vi "ABB Test Heat run.vi"(10 "Measure":enum16{"Full Load", "Partial Load", "No Load"}(ring), 11 "Heat run Type":enum16{"Full Load", "Partial- & No-Load"}(ring)) -> ()   [LabVIEW 2017]
uses:
  Temp error msg.ctl
  <vilib>/Analysis/baseanly.llb/Mean (DBL).vi
  ABB global.vi
  <vilib>/Analysis/NI_AALBase.lvlib
panel:
  in  "Temp error":T1="Error: Temperature measurement "
  out "Additional Temperatures 2":string[][](table)
  out "Bearing Run readings":string[][](table)
  in  "Rated":T2
  in  "copying":string="Copying.."
  in  "copy to bearing":bool
  in  "Averaging":i32=1 min=1 max=1000
  in  "Smooth power\n    readings":bool
  in  "Reading Category":T3(ring)=enum."Wdg Temp"
  out "Power Readings":string[][](table)
  in  "Comments":string
  in  "Start":bool
  out "Type of Run":string
  out "Additional Temperatures":string[][](table)
  in  "Stabilitymessg":string="Thermal Stability reached"
  out "Time to Next reading":dbl(slide) scale=0.0..30.0 scale format="%#.1f"
  out "Start Time":dbl
  out "Temperatures":string[][](table)
  out "Readings":string[][](table)
  out "saved Readings":dbl[][](array[numeric])
  out "Serial number":string
  out "W.O number":string
  out "Norma 5000 Error":string
  in  "Record":bool
  out "Readings Table":string[][](table)
  in  "View":enum16{"Graph", "Readings"}(ring)
  out "Number readings":i32
  out "Status":enum16{"Stopped", "Running", "Finished"}(ring)
  out "Timedate":string
  in  "End test":bool
  in  "Read Mode":enum16{"Auto", "Manual"}(ring)
  in  "Exit":bool
  out "Temperature Trend":cluster{dbl[], "Best Linear Fit":dbl[]}[](graph)
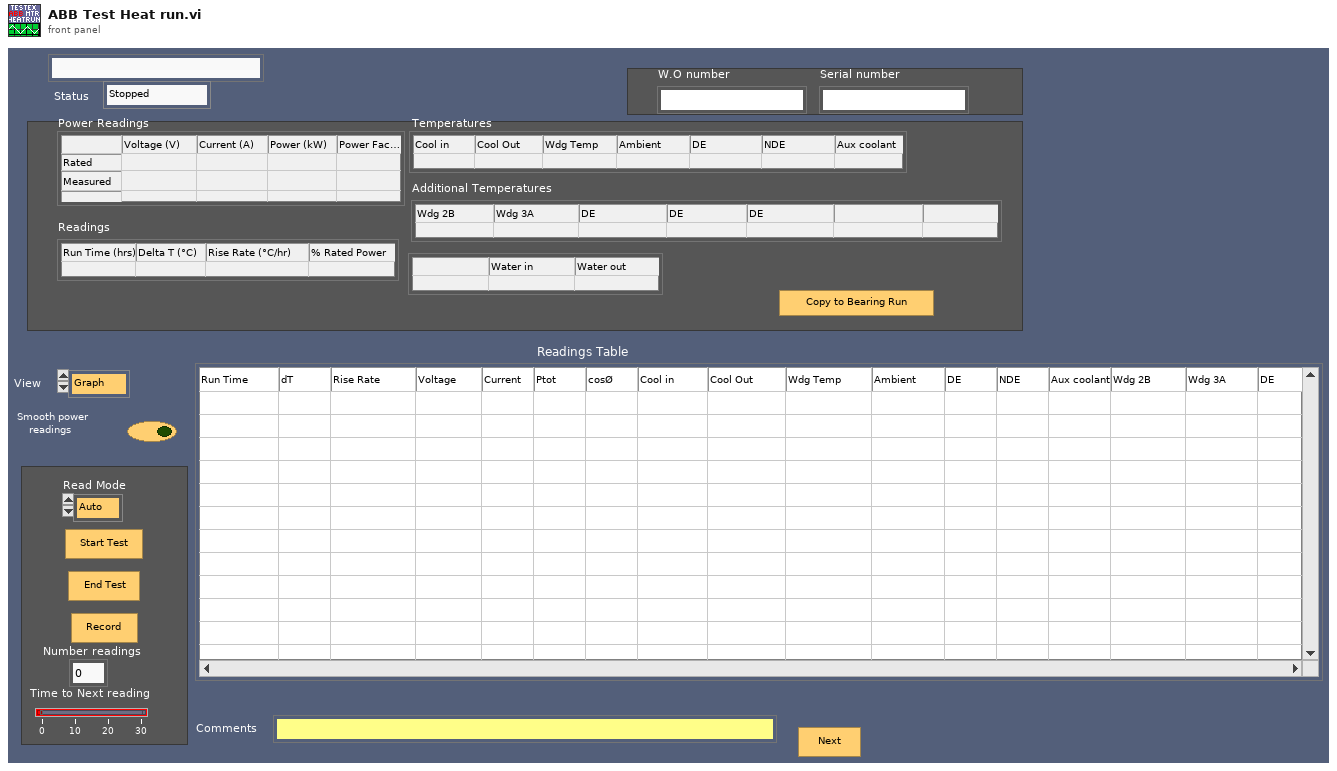
[diagram p1: front panel]
types:
  T1 = typedef "Temp error msg.ctl" = string
  T2 = cluster{"Voltage":dbl, "Current":dbl, "Power":dbl, "power factor":dbl}
  T3 = enum16{"None", "Cool in", "Cool Out", "Wdg Temp", "Ambient", "DE", "NDE", "Aux coolant"}
  T4 = enum16{"No load", "Locked Rotor", "Heat run", "NoLd heat run", "Partial heat run"}
  T5 = enum16{"Heat run", "Bearing run", "NoLd Heat Run", "Partial heat run"}
  T6 = cluster{"VT Primary":dbl, "VT Secondary":dbl, "CT  Primary":dbl, "CT Secondary":dbl, "Current Shunt":enum16{"Internal", "External"}, "Avg interval":dbl}
  T7 = cluster{"VT Primary":dbl, "VT Secondary":dbl, "CT  Primary":dbl, "CT Secondary":dbl, "Current Shunt":enum16{"Internal", "External"}, "Averaging interval (secs)":dbl}
  T8 = cluster{"Visa sesssion":refnum<visa-resource-name>, "error":errorcluster}
  T9 = cluster{"Simulate Norma":bool, "Norma 5000 Address":u8, "WebDaq IP Address":string, "Simulate cDAQ":bool}
  T10 = cluster{"Thermal Stability (deg/hr)":dbl, "Reading interval (mins)":dbl}
  T11 = cluster{"String":string, "String":string, "String":string, "String":string}
  T12 = cluster{"String":dbl, "String":dbl, "String":dbl, "String":dbl}
  T13 = cluster{"temp. alloc":i32[], "category":i32[], "Category names":string[], "Category none names":string[]}
  T14 = cluster{"V":dbl, "A":dbl, "W":dbl, "VA":dbl, "VAr":dbl, "Pf":dbl}
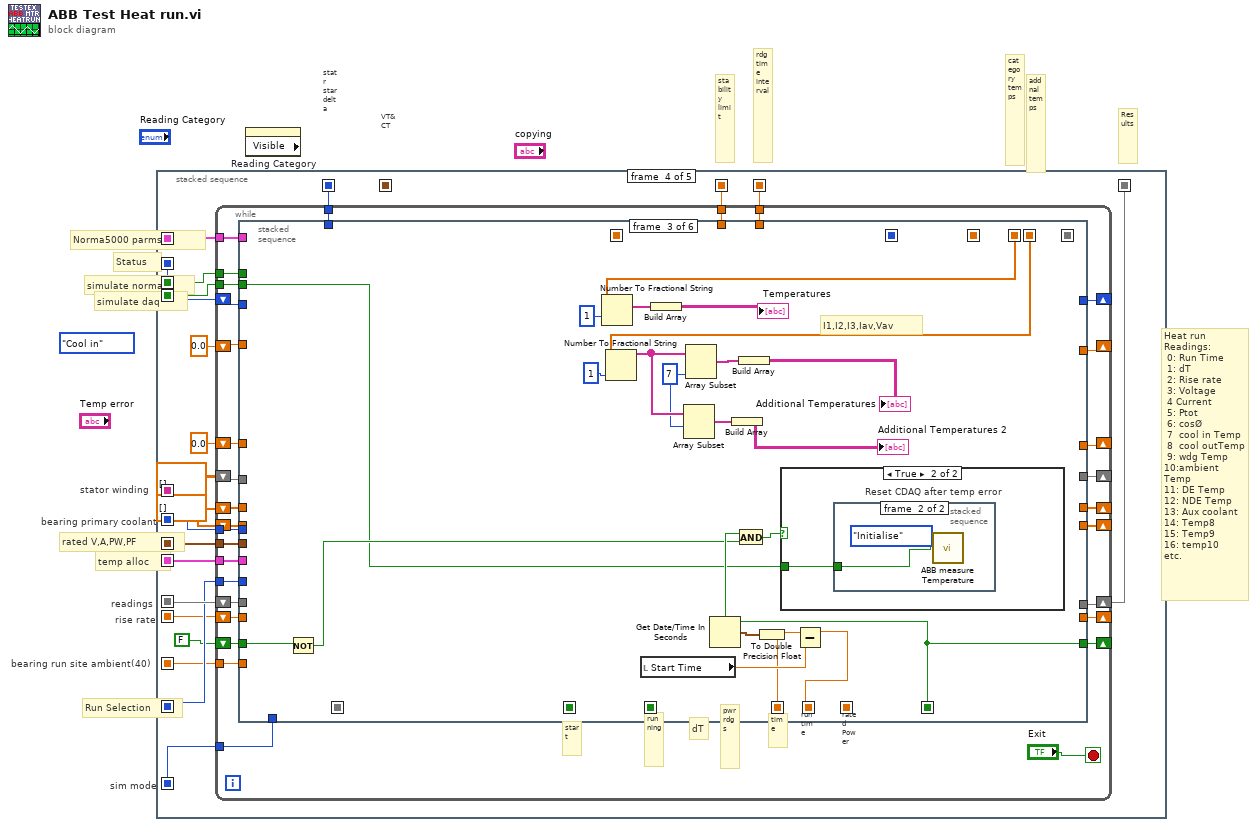
[diagram p0: block diagram]
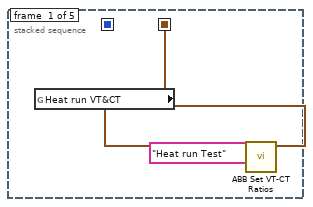
[diagram p2: hidden frame]
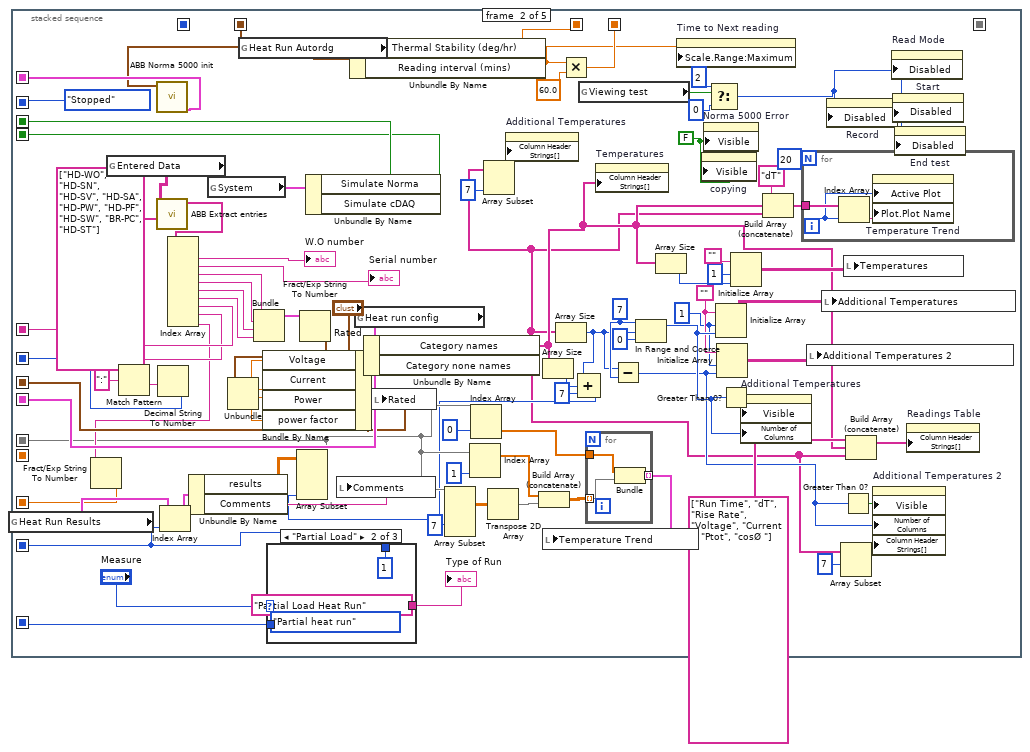
[diagram p3: hidden frame]
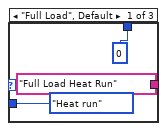
[diagram p4: hidden frame]
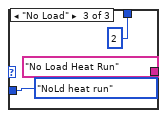
[diagram p5: hidden frame]
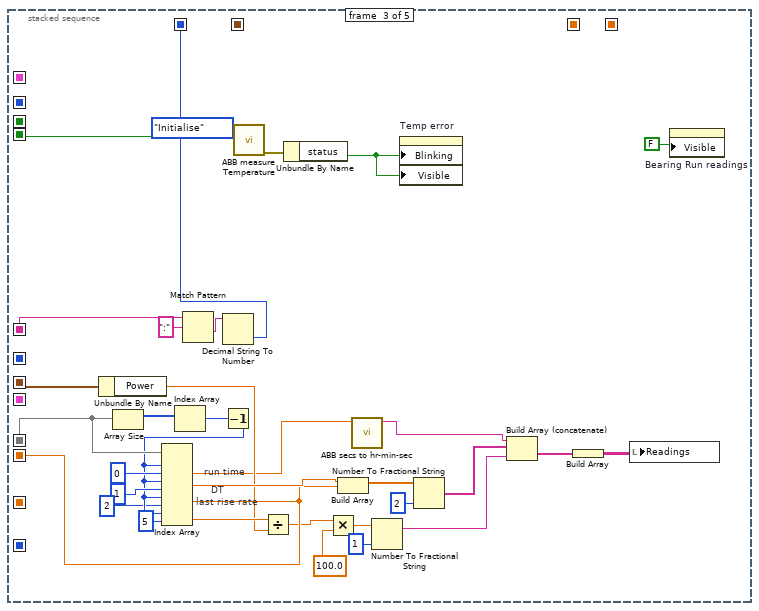
[diagram p6: hidden frame]
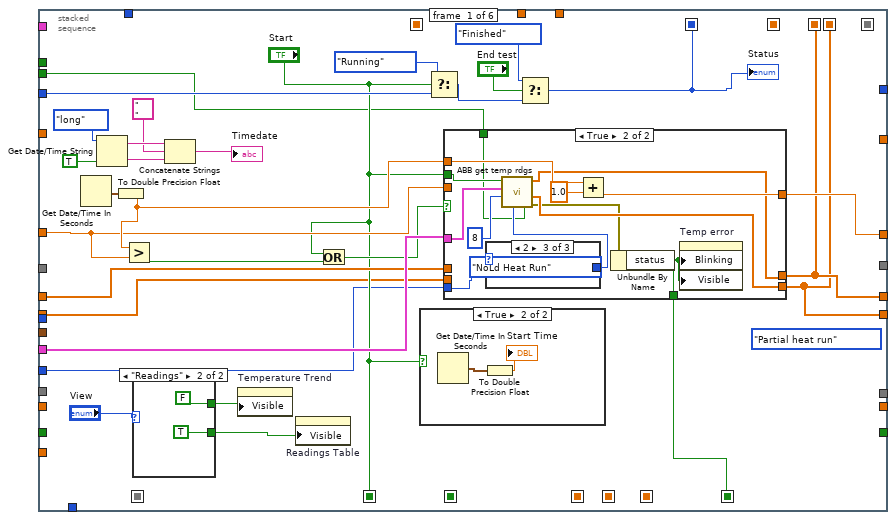
[diagram p7: hidden frame]
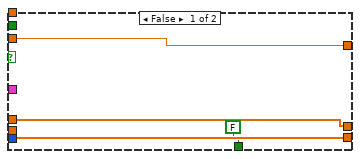
[diagram p9: hidden frame]
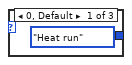
[diagram p10: hidden frame]
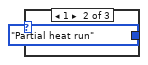
[diagram p11: hidden frame]
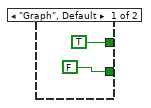
[diagram p12: hidden frame]
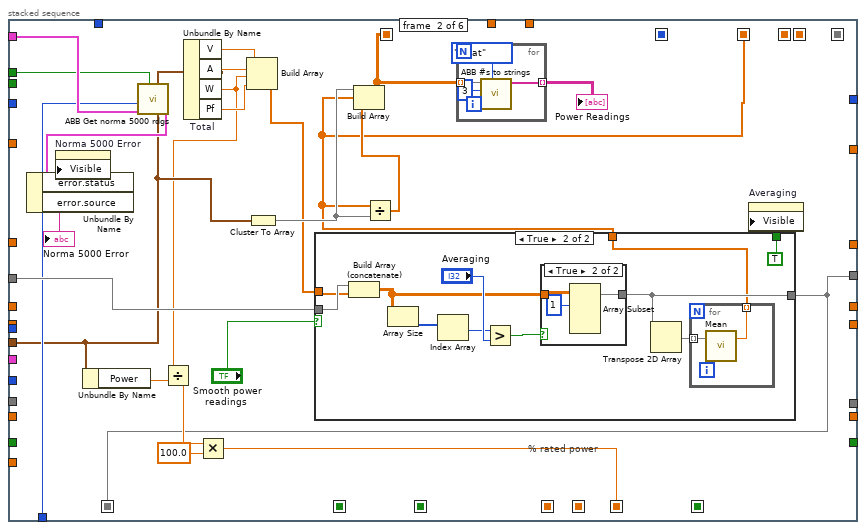
[diagram p13: hidden frame]
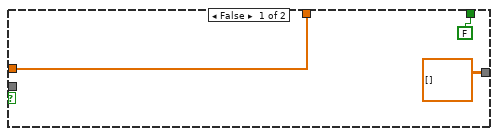
[diagram p14: hidden frame]
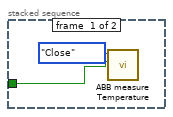
[diagram p17: hidden frame]
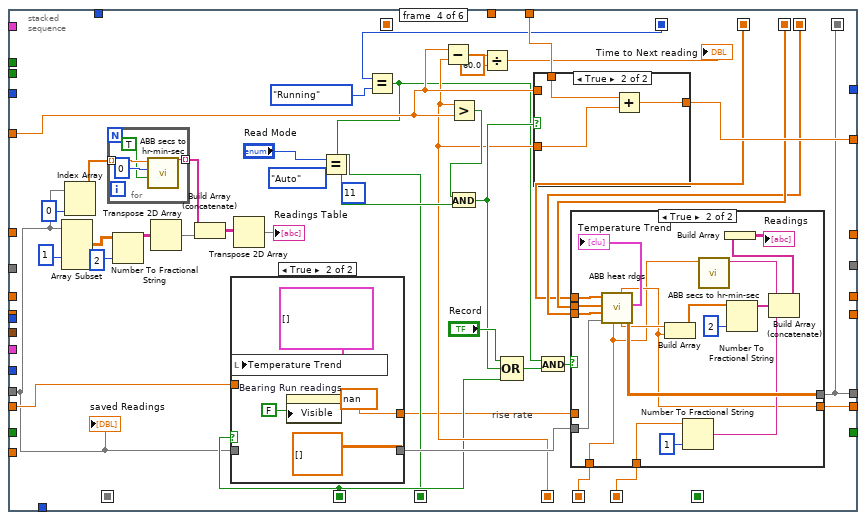
[diagram p18: hidden frame]
diagram:
  (unwired) T3."Cool in" ("Reading Category")
  # "bearing run site ambient(40)"
  # "bearing primary coolant"
  # "VT&CT"
  # "statr stardelta"
  # "stator winding"
  # "rise rate"
  # "readings"
  # "sim mode"
  # "simulate daq"
  # "addnal temps"
  # "category temps"
  # "Run Selection"
  # "stability limit"
  # "Results"
  # "rdg time interval"
  # "Heat run Readings:\n 0: Run Time\n 1: dT\n 2: Rise rate\n 3: Voltage\n 4 Current\n 5: Ptot\n 6: cosØ\n 7  cool in Temp\n 8  cool outTemp\n 9: wdg Temp\n10:ambient Temp\n11: DE Temp\n12: NDE Temp\n13: Aux coolant\n14: Temp8\n15: Temp9\n16: temp10\netc."
  # "temp alloc"
  # "rated V,A,PW,PF"
  # "simulate norma"
  # "Norma5000 parms"
  # "Status"
  n1 = stacked-sequence {
    seq-local: [_ enum16{"Stopped", "Running", "Finished"}."Stopped" ("Status") _ _ _] -> [_ _ _ w161 _]
    seq-local: [_ w90 _ _ _] -> [_ _ _ w160 w474]
    seq-local: [_ w88 _ _ _] -> [_ _ _ w159 w473]
    seq-local: [_ w38 _ _ _] -> [_ _ w129 w158 _]
    seq-local: [_ w7 _ _ _] -> [_ _ w138 w157 _]
    seq-local: [_ w53 _ _ _] -> [_ _ _ w155 _]
    seq-local: [_ w75 _ _ _] -> [_ _ _ w154 _]
    seq-local: [_ _ _ w152 _] -> [_ _ _ _ w471]
    seq-local: [_ w65 _ _ _] -> [_ _ _ w151 _]
    seq-local: [_ w47 _ _ _] -> [_ _ _ w148 w470]
    seq-local: [_ w51 _ _ _] -> [_ _ w110 w146 w467]
    seq-local: [_ w45 _ _ _] -> [_ _ _ w147 _]
    seq-local: [_ _ w132 _ _] -> [_ _ _ w145 _]
    seq-local: [_ w30 _ _ _] -> [_ _ w113 _ _]
    seq-local: [_ _ w112 _ _] -> [_ _ _ w144 _]
    seq-local: [w2 _ _ _ _] -> [_ w31 _ _ w469]
    seq-local: [_ w26 _ _ _] -> [_ _ _ w143 _]
    seq-local: [_ w24 _ _ _] -> [_ _ _ w142 _]
    frame #0 {
      n2 = global read "ABB global.vi" "Heat run VT&CT"() -> (w3:T6)
      n3 = call "ABB Set VT-CT Ratios.vi"("Test name"="Heat run Test", "VT and CT Ratios"=w3) -> ("VT and CT Ratios out"=w2:T7)  [unwired: 9 in]
    }
    frame #1 {
      w21 = 7 ("upper limit")
      w20 = ""
      w19 = 1 ("dimension size")
      w52 = FALSE ("Visible")
      n4 = global read "ABB global.vi" "Heat Run Results"() -> (w48:cluster{"results":dbl[][], "Comments":string}[])
      n5 = global read "ABB global.vi" "Entered Data"() -> (w71:string[][])
      n6 = call "ABB Norma 5000 init.vi"("VT and CT Ratios"=w31) -> ("norma 5000 parms out"=w90:T8)  [unwired: 10 in]
      n7 = call "ABB Extract entries.vi"("Entry IDs"=string[] ["HD-WO", "HD-SN", "HD-SV", "HD-SA", "HD-PW", "HD-PF", "HD-SW", "BR-PC", "HD-ST"], "Entry table in"=w71) -> ("Selected Entries"=w37:string[])  [unwired: 9 in]
      n8 = Index Array(array=w37) -> (element #1=→"W.O number":string, element #2=→"Serial number":string, element #3=w67:string, element #4=w55:string, element #5=w54:string, element #6=w56:string, element #7=w30:string, element #8=w27:string, element #9=w25:string)  [unwired: 9 in]
      n9 = Fract/Exp String To Number(string=w25) -> (number=w24:dbl)  [unwired: 3 in, 1 out]
      n10 = Match Pattern(string=w27, regular expression=":") -> (after substring=w28:string)  [unwired: 1 in, 3 out]
      n11 = Decimal String To Number(string=w28) -> (number=w26:i32)  [unwired: 2 in, 1 out]
      n12 = global read "ABB global.vi" "System"() -> (w89:T9)
      n13 = global read "ABB global.vi" "Heat Run Autordg"() -> (w87:T10)
      n14 = Bundle("String"=w67, "String"=w55, "String"=w54, "String"=w56) -> (w66:T11)  [unwired: 1 in]
      n15 = case shown="\"Partial Load\"" "Measure" {
        tunnel: ["Full Load Heat Run" "Partial Load Heat Run" "No Load Heat Run"] -> w50
        tunnel: [0 1 2] -> w47
        tunnel: [T4."Heat run" ("Simulate Mode") T4."Partial heat run" ("Simulate Mode") T4."NoLd heat run" ("Simulate Mode")] -> w45
        frame "Full Load", Default {
        }
        frame "Partial Load" {
        }
        frame "No Load" {
        }
      }
      "Type of Run" <- w50
      n16 = Index Array(array=w48, index=w47) -> (element=w61:cluster{"results":dbl[][], "Comments":string})
      n17 = Unbundle By Name(w61) -> ("results"=w8:dbl[][], "Comments"=w49:string)
      n18 = Fract/Exp String To Number(string=w66) -> (number=w43:T12)  [unwired: 3 in, 1 out]
      n19 = Unbundle(w43) -> ("String"=w42:dbl, "String"=w41:dbl, "String"=w40:dbl, "String"=w39:dbl)
      n20 = Bundle By Name(cluster="Rated", "Voltage"=w42, "Current"=w41, "Power"=w40, "power factor"=w39) -> (w38:T2)
      n21 = Unbundle By Name(w89) -> ("Simulate Norma"=w88:bool, "Simulate cDAQ"=w51:bool)
      n22 = local write "Comments"(w49) -> ()
      n23 = Unbundle By Name(w87) -> ("Thermal Stability (deg/hr)"=w65:dbl, "Reading interval (mins)"=w74:dbl)
      n24 = global read "ABB global.vi" "Heat run config"() -> (w53:T13)
      n25 = Unbundle By Name(w53) -> ("Category names"=w5:string[], "Category none names"=w4:string[])
      n26 = local write "Rated"(w38) -> ()
      n27 = Array Subset(array=w4, length=7) -> (w15:string[])  [unwired: 1 in]
      n28 = property on="Additional Temperatures" class="Tbl (strict)"("Column Header Strings[]"=w15) -> ()  [unwired: 2 in, 2 out]
      n29 = Array Size(array=w5) -> (size(s)=w11:i32)
      n30 = Array Size(array=w4) -> (size(s)=w10:i32)
      n31 = Multiply(x=w74, y=60.0) -> (x*y=w75:dbl)
      n32 = Compound Arithmetic op=ADD(w10, w11, 7 ("value")) -> (w6:i32)
      n33 = Array Subset(array=w8, length (col)=w6) -> (w7:dbl[][])  [unwired: 3 in]
      n34 = Array Subset(array=w7, index (col)=7 ("index")) -> (w78:dbl[][])  [unwired: 3 in]
      n35 = Index Array(array=w7, index (col)=1 ("disabled index (col)")) -> (element=w32:dbl[])  [unwired: 1 in]
      n36 = Index Array(array=w7, index (col)=0 ("disabled index (col)")) -> (element=w80:dbl[])  [unwired: 1 in]
      n37 = Transpose 2D Array(2D array=w78) -> (transposed array=w77:dbl[][])
      n38 = Build Array (concatenate)(w32, w77) -> (w33:dbl[][])
      n39 = global read "ABB global.vi" "Viewing test"() -> (w60:bool)
      n40 = for {
        tunnel: w80 -> [w103]
        tunnel: w33 -> [w102] mode=indexing
        tunnel: [w101] -> w76 mode=indexing
        n41 = Bundle(w103, w102) -> (w101:cluster{dbl[], dbl[]})  [unwired: 1 in]
      }
      n42 = local write "Temperature Trend"(w76) -> ()
      n43 = property on="Temperatures" class="Tbl (strict)"("Column Header Strings[]"=w5) -> ()  [unwired: 2 in, 2 out]
      n44 = Subtract(x=w10, y=w21) -> (x-y=w16:i32)
      n45 = In Range and Coerce(upper limit=w21, x=w10, lower limit=0) -> (coerced(x)=w23:i32)  [unwired: 1 out]
      n46 = Array Size(array=w5) -> (size(s)=w85:i32)
      n47 = property on="Time to Next reading" class="Slide (strict)"("Scale.Range:Maximum"=w74) -> ()  [unwired: 2 in, 2 out]
      n48 = property on="copying" class="Str"("Visible"=w52) -> ()  [unwired: 2 in, 2 out]
      n49 = property on="Norma 5000 Error" class="Str"("Visible"=w52) -> ()  [unwired: 2 in, 2 out]
      n50 = Select(t=2, s=w60, f=0) -> (s? t:f=w57:i32)
      n51 = Initialize Array(w20, w19, w23) -> (w64:string[][])
      n52 = Initialize Array(w20, w19, w16) -> (w18:string[][])
      n53 = Greater Than 0?(x=w23) -> (x > 0?=w63:bool)
      n54 = Initialize Array("", 1 ("dimension size"), w85) -> (w83:string[][])
      n55 = property on="Additional Temperatures" class="Tbl (strict)"("Visible"=w63, "Number of Columns"=w23) -> ()  [unwired: 2 in, 2 out]
      n56 = Build Array (concatenate)("dT", w5, w4) -> (w36:string[])
      n57 = for {
        N: 20 -> [_]
        tunnel: w36 -> [w106]
        i -> [w105]
        n58 = Index Array(array=w106, index=w105) -> (element=w104:string)
        n59 = property on="Temperature Trend" class="XYGraph (strict)"("Active Plot"=w105, "Plot.Plot Name"=w104) -> ()  [unwired: 2 in, 2 out]
      }
      n60 = local write "Additional Temperatures 2"(w18) -> ()
      n61 = local write "Additional Temperatures"(w64) -> ()
      n62 = property on="Record" class="Bool"("Disabled"=w57) -> ()  [unwired: 2 in, 2 out]
      n63 = Array Subset(array=w4, index=7) -> (w12:string[])  [unwired: 1 in]
      n64 = Greater Than 0?(x=w16) -> (x > 0?=w17:bool)
      n65 = local write "Temperatures"(w83) -> ()
      n66 = Build Array (concatenate)(string[] ["Run Time", "dT", "Rise Rate", "Voltage", "Current ", "Ptot", "cosØ "], w5, w4) -> (w72:string[])
      n67 = property on="Additional Temperatures 2" class="Tbl (strict)"("Visible"=w17, "Number of Columns"=w16, "Column Header Strings[]"=w12) -> ()  [unwired: 2 in, 2 out]
      n68 = property on="Read Mode" class="Enum (strict)"("Disabled"=w57) -> ()  [unwired: 2 in, 2 out]
      n69 = property on="Start" class="Bool"("Disabled"=w57) -> ()  [unwired: 2 in, 2 out]
      n70 = property on="End test" class="Bool"("Disabled"=w57) -> ()  [unwired: 2 in, 2 out]
      n71 = property on="Readings Table" class="Tbl (strict)"("Column Header Strings[]"=w72) -> ()  [unwired: 2 in, 2 out]
    }
    frame #2 {
      # "DT"
      # "run time"
      # "last rise rate"
      n72 = Unbundle By Name(w129) -> ("Power"=w128:dbl)
      n73 = Array Size(array=w138) -> (size(s)=w140:i32[])
      n74 = Index Array(array=w140) -> (element=w139:i32)  [unwired: 1 in]
      n75 = Match Pattern(string=w113, regular expression=":") -> (after substring=w114:string)  [unwired: 1 in, 3 out]
      n76 = Decimal String To Number(string=w114) -> (number=w112:i32)  [unwired: 2 in, 1 out]
      n77 = Decrement(x=w139) -> (x-1=w135:i32)
      n78 = Index Array(array=w138, index (row) #1=w135, index (col) #1=0, index (row) #2=w135, index (col) #2=1 ("disabled index (col)"), index (row) #3=w135, index (col) #3=2 ("disabled index (col)"), index (row) #4=w135, index (col) #4=5 ("disabled index (col)")) -> (element #1=w117:dbl, element #2=w134:dbl, element #3=w132:dbl, element #4=w130:dbl)
      n79 = call "ABB measure Temperature.vi"("Simulate"=w110, "Mode"=enum16{"Initialise", "Read", "Close"}."Initialise") -> ("error out"=w108:errorcluster)  [unwired: 7 in, 2 out]
      n80 = Divide(x=w130, y=w128) -> (x/y=w125:dbl)
      n81 = Unbundle By Name(w108) -> ("status"=w107:bool)
      n82 = Multiply(x=w125, y=100.0) -> (x*y=w119:dbl)
      n83 = Build Array(w134, w132) -> (w127:dbl[])
      n84 = call "ABB secs to hr-min-sec.vi"("Seconds"=w117) -> ("hr:min:secs"=w116:string)  [unwired: 10 in]
      n85 = Number To Fractional String(number=w119, precision (6)=i16 1) -> (F-format string=w122:string)  [unwired: 2 in]
      n86 = property on="Temp error" class="Str (strict)"("Blinking"=w107, "Visible"=w107) -> ()  [unwired: 2 in, 2 out]
      n87 = Number To Fractional String(number=w127, precision (6)=i16 2) -> (F-format string=w123:string[])  [unwired: 2 in]
      n88 = Build Array (concatenate)(w116, w123, w122) -> (w121:string[])
      n89 = Build Array(w121) -> (w120:string[][])
      n90 = local write "Readings"(w120) -> ()
      n91 = property on="Bearing Run readings" class="Tbl (strict)"("Visible"=FALSE) -> ()  [unwired: 2 in, 2 out]
    }
    frame #3 {
      w150 = dbl[] []
      n92 = while {
        shift-right: [w190] -> _
        shift-left: w161 -> [w191]
        tunnel: w160 -> [w189]
        tunnel: w159 -> [w188]
        tunnel: w158 -> [w187]
        shift-right: [w185] -> w152
        shift-left: w157 -> [w186]
        shift-right: [w182] -> _
        shift-left: 0.0 -> [w184]
        shift-right: [w183] -> _
        shift-left: w150 -> [w180]
        tunnel: w155 -> [w181]
        tunnel: w154 -> [w179]
        shift-right: [w177] -> _
        shift-left: 0.0 -> [w178]
        tunnel: w151 -> [w176]
        shift-right: [w174] -> _
        shift-left: w150 -> [w175]
        shift-right: [w172] -> _
        shift-left: dbl[][] [] -> [w173]
        tunnel: w148 -> [w171]
        tunnel: w147 -> [w170]
        tunnel: w146 -> [w169]
        shift-right: [w168] -> _
        shift-left: w145 -> [w167]
        tunnel: w144 -> [w166]
        tunnel: w143 -> [w165]
        tunnel: w142 -> [w164]
        shift-right: [w163] -> _
        shift-left: FALSE -> [w162]
        stop <- "Exit" stop-if-true
        # "run time"
        # "% rated Power"
        # "running"
        # "time"
        # "dT"
        # "pwr rdgs"
        # "start"
        n93 = stacked-sequence {
          seq-local: ["Start" _ _ _ _ _] -> [_ _ _ w346 _ _]
          seq-local: [_ w258 _ _ _ _] -> [_ _ _ w340 _ _]
          seq-local: [_ _ w316 _ _ _] -> [_ _ _ w351 _ _]
          seq-local: [w200 _ _ _ _ _] -> [_ _ _ w344 w402 _]
          seq-local: [w199 _ _ _ _ _] -> [_ _ w314 w343 _ _]
          seq-local: [_ _ _ w342 _ _] -> [_ _ _ _ w408 _]
          seq-local: [w196 _ _ _ _ _] -> [_ _ w312 w341 _ _]
          seq-local: [_ w262 _ _ _ _] -> [_ _ _ _ _ _]
          seq-local: [_ _ _ w339 _ _] -> [_ _ _ _ w401 w422]
          seq-local: [_ w250 _ _ _ _] -> [_ _ _ w337 _ _]
          seq-local: [_ w249 _ _ _ _] -> [_ _ _ _ _ _]
          seq-local: [_ _ w309 _ _ _] -> [_ _ _ w338 _ _]
          seq-local: [w193 _ _ _ _ _] -> [_ _ w303 _ _ _]
          tunnel: w191 -> [w216 _ _ _ w412 _]
          tunnel: [_ _ _ _ w402 _] -> w190
          tunnel: w189 -> [_ w274 _ _ _ _]
          tunnel: w188 -> [_ w270 _ _ _ _]
          tunnel: w187 -> [_ w255 _ _ _ _]
          tunnel: w186 -> [_ _ _ w332 w416 _]
          tunnel: [_ _ _ w339 _ _] -> w185
          tunnel: w184 -> [w206 _ _ _ _ _]
          tunnel: [w199 _ _ _ _ _] -> w183
          tunnel: [w205 _ _ _ _ _] -> w182
          tunnel: w181 -> [w204 _ _ _ _ _]
          tunnel: w180 -> [w203 _ _ _ _ _]
          tunnel: w179 -> [_ _ _ w362 _ _]
          tunnel: w178 -> [_ _ _ w352 _ _]
          tunnel: [_ _ _ w361 _ _] -> w177
          tunnel: w176 -> [_ _ _ _ w415 _]
          tunnel: w175 -> [w197 _ _ _ _ _]
          tunnel: [w196 _ _ _ _ _] -> w174
          tunnel: w173 -> [_ w261 _ _ _ _]
          tunnel: [_ w249 _ _ _ _] -> w172
          tunnel: w171 -> [w195 _ _ _ _ _]
          tunnel: w170 -> [_ w256 _ _ _ _]
          tunnel: w169 -> [w194 _ w299 _ _ _]
          tunnel: [_ _ _ w336 _ _] -> w168
          tunnel: w167 -> [_ _ _ w335 w404 _]
          tunnel: w166 -> [_ _ _ _ _ _]
          tunnel: w165 -> [_ _ _ _ _ w421]
          tunnel: w164 -> [_ _ _ _ _ w420]
          tunnel: [_ _ w303 _ _ _] -> w163
          tunnel: w162 -> [_ _ w302 _ _ _]
          frame #0 {
            (unwired) T5."Partial heat run" ("sim type")
            n94 = Get Date/Time In Seconds() -> (seconds since 1Jan1904=w208:timestamp)
            n95 = Get Date/Time String(date format (0)=enum16{"short", "long", "abbreviated"}."long", want seconds? (F)=TRUE) -> (date string=w220:string, time string=w219:string)  [unwired: 1 in]
            n96 = To Double Precision Float(number=w208) -> (double precision float=w207:dbl)
            n97 = Greater?(x=w207, y=w206) -> (0:w202:bool)
            n98 = case shown="\"Readings\"" "View" {
              tunnel: [TRUE FALSE] -> w210
              tunnel: [FALSE TRUE] -> w209
              frame "Graph", Default {
              }
              frame "Readings" {
              }
            }
            n99 = Concatenate Strings(w220, "   ", w219) -> (→"Timedate":string)
            n100 = property on="Temperature Trend" class="XYGraph (strict)"("Visible"=w210) -> ()  [unwired: 2 in, 2 out]
            n101 = property on="Readings Table" class="Tbl (strict)"("Visible"=w209) -> ()  [unwired: 2 in, 2 out]
            n102 = Or(x="Start", y=w202) -> (x .or. y?=w201:bool)
            n103 = case shown="True" "Start" {
              frame False {
              }
              frame True {
                n104 = Get Date/Time In Seconds() -> (seconds since 1Jan1904=w224:timestamp)
                n105 = To Double Precision Float(number=w224) -> (double precision float=→"Start Time":dbl)
              }
            }
            n106 = Select(t=enum16{"Stopped", "Running", "Finished"}."Running", s="Start", f=w216) -> (s? t:f=w214:enum16{"Stopped", "Running", "Finished"})
            n107 = case shown="True" w201 {
              tunnel: w207 -> [_ w241]
              tunnel: [w228 w239] -> w205
              tunnel: w206 -> [w228 _]
              tunnel: w194 -> [_ w231]
              tunnel: w204 -> [_ w237]
              tunnel: [w227 w236] -> w199
              tunnel: w203 -> [w227 _]
              tunnel: "Start" -> [_ w238]
              tunnel: w197 -> [w226 _]
              tunnel: [w226 w235] -> w196
              tunnel: w195 -> [_ w233]
              tunnel: [FALSE ("status") w229] -> w193
              frame False {
              }
              frame True {
                n108 = case shown="2" w233 {
                  tunnel: [T5."Heat run" ("sim type") T5."Partial heat run" ("sim type") T5."NoLd Heat Run" ("sim type")] -> w232
                  frame 0, Default {
                  }
                  frame 1 {
                  }
                  frame 2 {
                  }
                }
                n109 = call "ABB get temp rdgs.vi"("Sim daq"=w231, "sim type"=w232, "# categories"=8, "run config"=w237, "start"=w238) -> ("error out"=w230:errorcluster, "Category none rdgs"=w235:dbl[], "Category rdgs"=w236:dbl[])  [unwired: 3 in, 1 out]
                n110 = Add(x=w241, y=1.0) -> (x+y=w239:dbl)
                n111 = Unbundle By Name(w230) -> ("status"=w229:bool)
                n112 = property on="Temp error" class="Str (strict)"("Blinking"=w229, "Visible"=w229) -> ()  [unwired: 2 in, 2 out]
              }
            }
            n113 = Select(t=enum16{"Stopped", "Running", "Finished"}."Finished", s="End test", f=w214) -> (s? t:f=w200:enum16{"Stopped", "Running", "Finished"})
            "Status" <- w200
          }
          frame #1 {
            # "% rated power"
            n114 = Unbundle By Name(w255) -> ("Power"=w254:dbl)
            n115 = call "ABB Get norma 5000 rdgs.vi"("Rated"=w255, "simulate"=w270, "norma 5000 parms in"=w274, "Simulate Mode"=w256) -> ("norma 5000 parms out"=w271:T8, "Total"=w269:T14)  [unwired: 3 in, 3 out]
            n116 = Unbundle By Name(w271) -> ("error.status"=w273:bool, "error.source"=→"Norma 5000 Error":string)
            n117 = property on="Norma 5000 Error" class="Str"("Visible"=w273) -> ()  [unwired: 2 in, 2 out]
            n118 = Unbundle By Name "Total"(w269) -> ("V"=w265:dbl, "A"=w264:dbl, "W"=w253:dbl, "Pf"=w263:dbl)
            n119 = Divide(x=w253, y=w254) -> (x/y=w252:dbl)
            n120 = Multiply(x=w252, y=100.0) -> (x*y=w250:dbl)
            n121 = Build Array(w265, w264, w253, w263) -> (w259:dbl[])
            n122 = Cluster To Array(cluster=w255) -> (array=w266:dbl[])
            n123 = case shown="True" "Smooth power\n    readings" {
              tunnel: w261 -> [_ w282]
              tunnel: w259 -> [w277 w281]
              tunnel: [dbl[][] [] w284] -> w249
              tunnel: [w277 w283] -> w258
              tunnel: [FALSE TRUE] -> w257
              frame False {
              }
              frame True {
                n124 = Build Array (concatenate)(w282, w281) -> (w285:dbl[][])
                n125 = Array Size(array=w285) -> (size(s)=w288:i32[])
                n126 = Index Array(array=w288) -> (element=w278:i32)  [unwired: 1 in]
                n127 = Greater?(x=w278, y="Averaging") -> (0:w286:bool)
                n128 = case shown="True" w286 {
                  tunnel: w285 -> [w291 w294]
                  tunnel: [w291 w293] -> w284
                  frame False {
                  }
                  frame True {
                    n129 = Array Subset(array=w294, index (row)=1 ("index")) -> (w293:dbl[][])  [unwired: 3 in]
                  }
                }
                n130 = Transpose 2D Array(2D array=w284) -> (transposed array=w280:dbl[][])
                n131 = for {
                  tunnel: w280 -> [w290] mode=indexing
                  tunnel: [w289] -> w283 mode=indexing
                  n132 = call-poly <vilib>:"Mean.vi"("X"=w290) -> ("mean"=w289:dbl)  [unwired: 1 out]
                }
              }
            }
            n133 = Divide(x=w258, y=w266) -> (x/y=w267:dbl[])
            n134 = Build Array(w266, w258, w267) -> (w262:dbl[][])
            n135 = for {
              tunnel: w262 -> [w298] mode=indexing
              tunnel: [w295] -> w268 mode=indexing
              n136 = call "ABB #s to strings.vi"("# type"=enum16{"Float", "Relative time HH:MM"}."Float", "Precision"=3, "Numbers in"=w298) -> ("Strings out"=w295:string[])  [unwired: 8 in]
            }
            "Power Readings" <- w268
            n137 = property on="Averaging" class="DigNum (strict)"("Visible"=w257) -> ()  [unwired: 2 in, 2 out]
          }
          frame #2 {
            w304 = 7 ("length")
            # "I1,I2,I3,Iav,Vav"
            n138 = Not(x=w302) -> (.not. x?=w300:bool)
            n139 = Number To Fractional String(number=w314, precision (6)=i16 1) -> (F-format string=w313:string[])  [unwired: 2 in]
            n140 = Number To Fractional String(number=w312, precision (6)=i16 1) -> (F-format string=w307:string[])  [unwired: 2 in]
            n141 = local read "Start Time"() -> (w317:dbl)
            n142 = Build Array(w313) -> (→"Temperatures":string[][])
            n143 = Array Subset(array=w307, index=w304) -> (w305:string[])  [unwired: 1 in]
            n144 = Array Subset(array=w307, length=w304) -> (w308:string[])  [unwired: 1 in]
            n145 = Get Date/Time In Seconds() -> (seconds since 1Jan1904=w318:timestamp)
            n146 = Build Array(w305) -> (→"Additional Temperatures 2":string[][])
            n147 = And(x=w303, y=w300) -> (x .and. y?=w301:bool)
            n148 = Build Array(w308) -> (→"Additional Temperatures":string[][])
            n149 = To Double Precision Float(number=w318) -> (double precision float=w316:dbl)
            n150 = case shown="True" w301 {
              tunnel: w299 -> [_ w320]
              frame False {
              }
              frame True {
                # "Reset CDAQ after temp error"
                n151 = stacked-sequence {
                  tunnel: w320 -> [w321 w323]
                  frame #0 {
                    n152 = call "ABB measure Temperature.vi"("Simulate"=w321, "Mode"=enum16{"Initialise", "Read", "Close"}."Close") -> ()  [unwired: 7 in, 3 out]
                  }
                  frame #1 {
                    n153 = call "ABB measure Temperature.vi"("Simulate"=w323, "Mode"=enum16{"Initialise", "Read", "Close"}."Initialise") -> ()  [unwired: 7 in, 3 out]
                  }
                }
              }
            }
            n154 = Subtract(x=w316, y=w317) -> (x-y=w309:dbl)
          }
          frame #3 {
            (unwired) 11 ("index")
            # "rise rate"
            n155 = Array Subset(array=w332, index (col)=1 ("index")) -> (w333:dbl[][])  [unwired: 3 in]
            n156 = Index Array(array=w332, index (col)=0 ("disabled index (col)")) -> (element=w331:dbl[])  [unwired: 1 in]
            n157 = for {
              tunnel: w331 -> [w368] mode=indexing
              tunnel: [w366] -> w327 mode=indexing
              n158 = call "ABB secs to hr-min-sec.vi"("round off secs"=TRUE, "Precision"=i16 0, "Seconds"=w368) -> ("hr:min:secs"=w366:string)  [unwired: 8 in]
            }
            n159 = Number To Fractional String(number=w333, precision (6)=i16 2) -> (F-format string=w347:string[][])  [unwired: 2 in]
            n160 = Transpose 2D Array(2D array=w347) -> (transposed array=w326:string[][])
            n161 = Build Array (concatenate)(w327, w326) -> (w330:string[][])
            n162 = case shown="True" w346 {
              tunnel: w332 -> [w374 _]
              tunnel: [w374 dbl[][] []] -> w355
              tunnel: w335 -> [w373 _]
              tunnel: [w373 nan] -> w334
              frame False {
              }
              frame True {
                n163 = local write "Temperature Trend"(cluster{dbl[], "Best Linear Fit":dbl[]}[] [] ("Temperature Trend")) -> ()
                n164 = property on="Bearing Run readings" class="Tbl (strict)"("Visible"=FALSE) -> ()  [unwired: 2 in, 2 out]
              }
            }
            n165 = Transpose 2D Array(2D array=w330) -> (transposed array=→"Readings Table":string[][])
            n166 = Equal?(x="Read Mode", y=enum16{"Auto", "Manual"}."Auto") -> (x = y?=w358:bool)
            n167 = Equal?(x=w344, y=enum16{"Stopped", "Running", "Finished"}."Running" ("x")) -> (x = y?=w342:bool)
            n168 = Subtract(x=w352, y=w351) -> (x-y=w350:dbl)
            n169 = Greater?(x=w351, y=w352) -> (0:w357:bool)
            n170 = And(x=w357, y=w358) -> (x .and. y?=w356:bool)
            n171 = Divide(x=w350, y=60.0) -> (x/y=→"Time to Next reading":dbl)
            n172 = Compound Arithmetic op=OR("Record", w356, w346) -> (w353:bool)
            n173 = case shown="True" w356 {
              tunnel: w362 -> [_ w371]
              tunnel: w351 -> [_ w372]
              tunnel: [w369 w370] -> w361
              tunnel: w352 -> [w369 _]
              frame False {
              }
              frame True {
                n174 = Add(x=w371, y=w372) -> (x+y=w370:dbl)
              }
            }
            n175 = And(x=w342, y=w353) -> (x .and. y?=w354:bool)
            n176 = case shown="True" w354 {
              tunnel: w355 -> [w380 w395]
              tunnel: [w380 w394] -> w339
              tunnel: w340 -> [_ w398]
              tunnel: w343 -> [_ w397]
              tunnel: w341 -> [_ w393]
              tunnel: w338 -> [_ w381]
              tunnel: w337 -> [_ w382]
              tunnel: [w379 w383] -> w336
              tunnel: w334 -> [w379 _]
              frame False {
              }
              frame True {
                n177 = call "ABB heat rdgs.vi"("Run Time"=w381, "Readings in"=w395, "Addnl temps"=w393, "temperatures"=w397, "power"=w398) -> ("Readings out"=w394:dbl[][], "Temperature trend"=→"Temperature Trend":cluster{dbl[], dbl[]}[], "dT"=w386:dbl, "rise rate"=w383:dbl)  [unwired: 3 in]
                n178 = Build Array(w386, w383) -> (w390:dbl[])
                n179 = Number To Fractional String(number=w382, precision (6)=i16 1) -> (F-format string=w384:string)  [unwired: 2 in]
                n180 = call "ABB secs to hr-min-sec.vi"("Seconds"=w381) -> ("hr:min:secs"=w388:string)  [unwired: 10 in]
                n181 = Number To Fractional String(number=w390, precision (6)=i16 2) -> (F-format string=w392:string[])  [unwired: 2 in]
                n182 = Build Array (concatenate)(w388, w392, w384) -> (w391:string[])
                n183 = Build Array(w391) -> (→"Readings":string[][])
              }
            }
            "saved Readings" <- w332
          }
          frame #4 {
            n184 = Array Size(array=w416) -> (size(s)=w419:i32[])
            n185 = Index Array(array=w419) -> (element=w418:i32)  [unwired: 1 in]
            n186 = Not Equal?(x=w412, y=enum16{"Stopped", "Running", "Finished"}."Stopped") -> (x != y?=w410:bool)
            n187 = Greater?(x=w418, y=2) -> (0:w413:bool)
            n188 = Absolute Value(x=w404) -> (abs(x)=w403:dbl)
            n189 = Less?(x=w403, y=w415) -> (x < y?=w414:bool)
            n190 = Wait Until Next ms Multiple(millisecond multiple=u32 200) -> ()  [unwired: 1 out]
            n191 = Compound Arithmetic op=AND(w414, w410, w413) -> (w407:bool)
            n192 = And(x=w407, y=w408) -> (x .and. y?=w406:bool)
            n193 = Select(t=enum16{"Stopped", "Running", "Finished"}."Finished", s=w406, f=w402) -> ()  [unwired: 1 out]
            n194 = property on="Stabilitymessg" class="Str"("Visible"=w407, "Blinking"=w407) -> ()  [unwired: 2 in, 2 out]
            n195 = property on="Time to Next reading" class="Slide (strict)"("Visible"=w408) -> ()  [unwired: 2 in, 2 out]
            n196 = Array Size(array=w401) -> (size(s)=w400:i32[])
            n197 = Index Array(array=w400) -> (element=→"Number readings":i32)  [unwired: 1 in]
          }
          frame #5 {
            n198 = case shown="True" "copy to bearing" {
              tunnel: w422 -> [_ w426]
              tunnel: w421 -> [_ w425]
              tunnel: w420 -> [_ w424]
              frame False {
              }
              frame True {
                n199 = stacked-sequence {
                  tunnel: w426 -> [_ w456 _]
                  tunnel: w425 -> [_ w448 _]
                  tunnel: w424 -> [_ w442 _]
                  frame #0 {
                    w427 = TRUE ("Visible")
                    n200 = property on="copying" class="Str"("Visible"=w427) -> ()  [unwired: 2 in, 2 out]
                    n201 = property on="Bearing Run readings" class="Tbl (strict)"("Visible"=w427) -> ()  [unwired: 2 in, 2 out]
                  }
                  frame #1 {
                    w430 = 2
                    (unwired) nan
                    # "Bearing run Readings:\n 0: Run Time\n 1: DE Rise\n 2: NDE Rise\n 3:DT\n4: Cool In\n5:Ambient\n6:DE Temp\n8: NDE Temp\n9: temp\netc."
                    # "Ambient"
                    # "Aux coolant"
                    # "NDE"
                    # "DE"
                    # "Run time"
                    n202 = Index Array(array=w456, index (col) #1=0 ("disabled index (col)"), index (col) #2=11 ("index (col)"), index (col) #3=12 ("index (col)"), index (col) #4=13 ("index (col)"), index (col) #5=10 ("index (col)")) -> (element #1=w450:dbl[], element #2=w445:dbl[], element #3=w444:dbl[], element #4=w447:dbl[], element #5=w446:dbl[])  [unwired: 5 in]
                    n203 = Build Array(w447, w446, w445, w444) -> (w443:dbl[][])
                    n204 = Transpose 2D Array(2D array=w443) -> (transposed array=w431:dbl[][])
                    n205 = for {
                      tunnel: w450 -> [w460] mode=indexing
                      tunnel: w446 -> [_] mode=indexing
                      tunnel: w448 -> [w465]
                      tunnel: w431 -> [w464] mode=indexing
                      tunnel: w442 -> [w463]
                      shift-right: [w462] -> w440
                      shift-left: dbl[][] [] ("Readings out") -> [w461]
                      tunnel: [w460] -> w437
                      tunnel: [w459] -> w439
                      tunnel: [w458] -> w438
                      tunnel: [w457] -> w428
                      n206 = call "ABB bearing rdgs.vi"("Run Time"=w460, "Site ambient"=w463, "Readings in"=w461, "temperatures"=w464, "Primary coolant"=w465) -> ("Readings out"=w462:dbl[][], "NDE rise"=w458:dbl, "DE rise"=w459:dbl, "rise rate"=w457:dbl)  [unwired: 2 in, 1 out]
                    }
                    n207 = Number To Fractional String(number=w439, precision (6)=w430) -> (F-format string=w435:string)  [unwired: 2 in]
                    n208 = Number To Fractional String(number=w428, precision (6)=w430) -> (F-format string=w429:string)  [unwired: 2 in]
                    n209 = Number To Fractional String(number=w438, precision (6)=w430) -> (F-format string=w434:string)  [unwired: 2 in]
                    n210 = call "ABB secs to hr-min-sec.vi"("Seconds"=w437) -> ("hr:min:secs"=w436:string)  [unwired: 10 in]
                    n211 = Wait (ms)(milliseconds to wait=u32 1000 ("millisecond timer value")) -> ()  [unwired: 1 out]
                    n212 = global write "ABB global.vi" "Bearing run results"(w440) -> ()
                    n213 = Build Array(w436, w435, w434, w429) -> (w433:string[])
                    n214 = Build Array(w433) -> (→"Bearing Run readings":string[][])
                  }
                  frame #2 {
                    n215 = property on="copying" class="Str"("Visible"=FALSE) -> ()  [unwired: 2 in, 2 out]
                  }
                }
              }
            }
          }
        }
      }
    }
    frame #4 {
      n216 = global read "ABB global.vi" "Viewing test"() -> (w472:bool)
      n217 = case shown="False" w473 {
        tunnel: w474 -> [w500 _]
        frame False {
          n218 = Unbundle By Name(w500) -> ("Visa sesssion"=w499:refnum<visa-resource-name>, "error"=w498:errorcluster)
          n219 = call "LNOPA01 Error Query.vi"("error in (no error)"=w498, "VISA session"=w499) -> ("error out"=w501:errorcluster, "dup VISA session"=w502:refnum<visa-resource-name>)  [unwired: 6 in, 2 out]
          n220 = call "LNOPA01 Close.vi"("error in (no error)"=w501, "VISA session"=w502) -> ("error out"=w503:errorcluster)  [unwired: 9 in]
          n221 = call <vilib>:"Simple Error Handler.vi"("error in (no error)"=w503) -> ()  [unwired: 4 in, 5 out]
        }
        frame True {
        }
      }
      n222 = call "ABB measure Temperature.vi"("Simulate"=w467, "Mode"=enum16{"Initialise", "Read", "Close"}."Close") -> ()  [unwired: 7 in, 3 out]
      n223 = case shown="False" w472 {
        tunnel: w471 -> [w480 _]
        tunnel: w470 -> [w478 _]
        tunnel: w469 -> [w475 _]
        frame False {
          n224 = global read "ABB global.vi" "Current test"() -> (w479:path)
          n225 = Two Button Dialog(message="Save results?", 1:"Discard" ("F button name (\"Cancel\")"), 2:"Save" ("T button name (\"OK\")")) -> (T button?=w481:bool)
          n226 = case shown="True" w481 {
            tunnel: w480 -> [_ w486]
            tunnel: w479 -> [_ w485]
            tunnel: w478 -> [_ w484]
            tunnel: w475 -> [_ w483]
            frame False {
            }
            frame True {
              n227 = stacked-sequence {
                tunnel: w486 -> [w493 _]
                tunnel: w485 -> [_ w496]
                tunnel: w484 -> [w490 _]
                tunnel: w483 -> [w487 _]
                frame #0 {
                  n228 = global write "ABB global.vi" "Heat run VT&CT"(w487) -> ()
                  n229 = global read "ABB global.vi" "Heat Run Results"() -> (w489:cluster{"results":dbl[][], "Comments":string}[])
                  n230 = global write "ABB global.vi" "Heat run Type"("Heat run Type") -> ()
                  n231 = Index Array(array=w489, index=w490) -> (element=w492:cluster{"results":dbl[][], "Comments":string})
                  n232 = Bundle By Name(cluster=w492, "results"=w493, "Comments"="Comments") -> (w495:cluster{"results":dbl[][], "Comments":string})
                  n233 = Replace Array Subset(array=w489, new element=w495, index=w490) -> (w491:cluster{"results":dbl[][], "Comments":string}[])
                  n234 = global write "ABB global.vi" "Heat Run Results"(w491) -> ()
                }
                frame #1 {
                  n235 = call "ABB Load-Save results.vi"("Path"=w496, "Mode"=enum16{"LOAD", "Save"}."Save") -> ()  [unwired: 10 in]
                }
              }
            }
          }
        }
        frame True {
        }
      }
    }
  }
  n236 = property on="Reading Category" class="Enum (strict)" props=["Visible"]() -> ()  [unwired: 2 in, 3 out]
